vi "Format Entry.vi"(8 "error in (no error)":errorcluster, 10 "Log Data":T1={"Time"=timestamp(0 s since 1904-01-01), "Level"=enum."INFO", "Logger"="", "Message"="", "Arguments"=[]} {"Time" format="%<%x %.3X>T"}, 11 "Simple in":refnum<class "SimpleLayout.lvclass">) -> (0 "error out":errorcluster, 2 "Log Entry":string, 3 "Simple out":refnum<class "SimpleLayout.lvclass">)   [LabVIEW 2019, in "TSC Event Logger.lvlib" / "SimpleLayout.lvclass"]
uses:
  SimpleLayout.lvclass
  Log Data.ctl
  Log/Event Level.ctl
  Layout.lvclass
  TSC Event Logger.lvlib
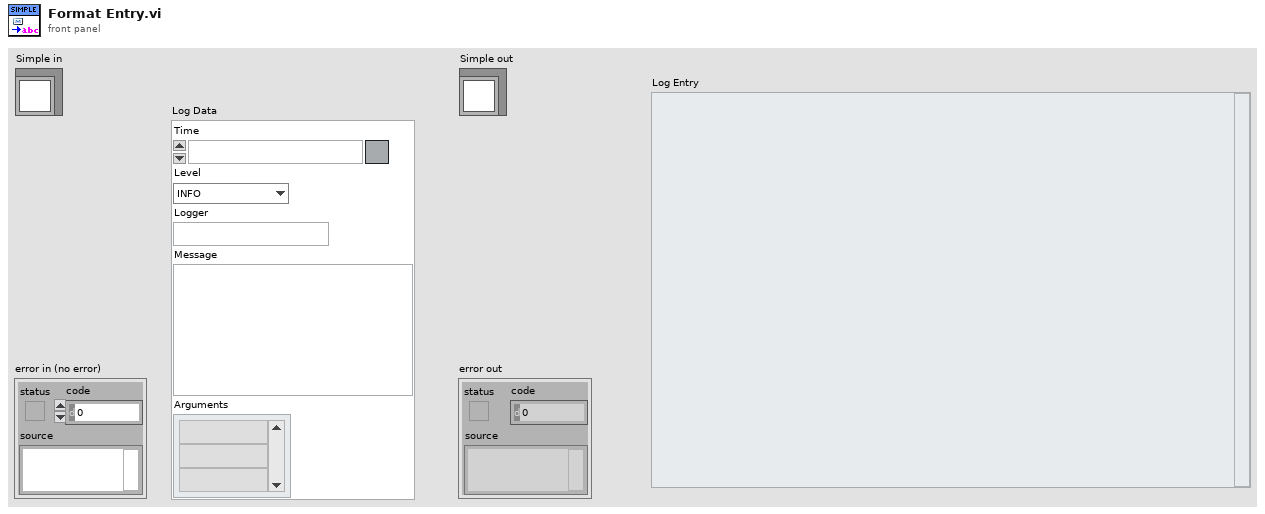
[diagram p1: front panel]
types:
  T1 = typedef "TSC Event Logger.lvlib/Log Data.ctl" = cluster{"Time":timestamp, "Level":T2, "Logger":string, "Message":string, "Arguments":string[]}
  T2 = typedef "TSC Event Logger.lvlib/Event Level.ctl" = enum16{"OFF", "TRACE", "DEBUG", "INFO", "WARN", "ERROR", "FATAL"}
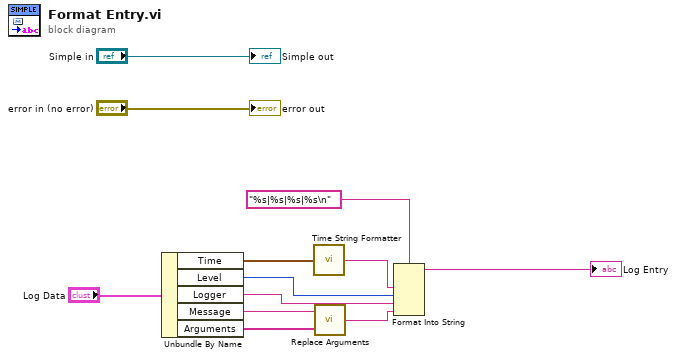
[diagram p0: block diagram]
diagram:
  n1 = Unbundle By Name("Log Data") -> ("Time"=w5:timestamp, "Level"=w9:T2, "Logger"=w8:string, "Message"=w3:string, "Arguments"=w2:string[])
  n2 = call "Time String Formatter.vi"("Time"=w5) -> ("Time string"=w4:string)
  n3 = call "Replace Arguments.vi"("Arguments"=w2, "Message"=w3) -> ("Output Message"=w1:string)
  n4 = Format Into String(format string="%s|%s|%s|%s\n", w4, w9, w8, w1) -> (resulting string=→"Log Entry":string)  [unwired: 2 in, 1 out]
  "error out" <- "error in (no error)"
  "Simple out" <- "Simple in"
